vi "graph_diag.vi"(4 "dt":dbl, 6 "Array in":dbl[](array[numeric]), 7 "Averaged":cluster{"xi used":dbl[], "yi":dbl[]}, 9 "DC(V)":dbl, 10 "LD Timetrace in":dbl[][](array[numeric]), 11 "dt":dbl) -> (2 "Time Domain Signal":cluster{"xi used":dbl[], "yi":dbl[]}[](graph), 3 "Spectra":cluster{"f0":dbl, "df":dbl, "magnitude":dbl[]}[](array[cluster]))   [LabVIEW 2013]
uses:
  <vilib>/express/express analysis/Spectral/Block/exnSpectralBlock spectral measurements RMS poly.vi
  <vilib>/express/express analysis/Spectral/Block/exnSpectralBlock spectral measurements RMS WFM.vi
  <vilib>/express/express analysis/Spectral/XNode/ExpressSpectralMeasurementsBlockNode.xnode
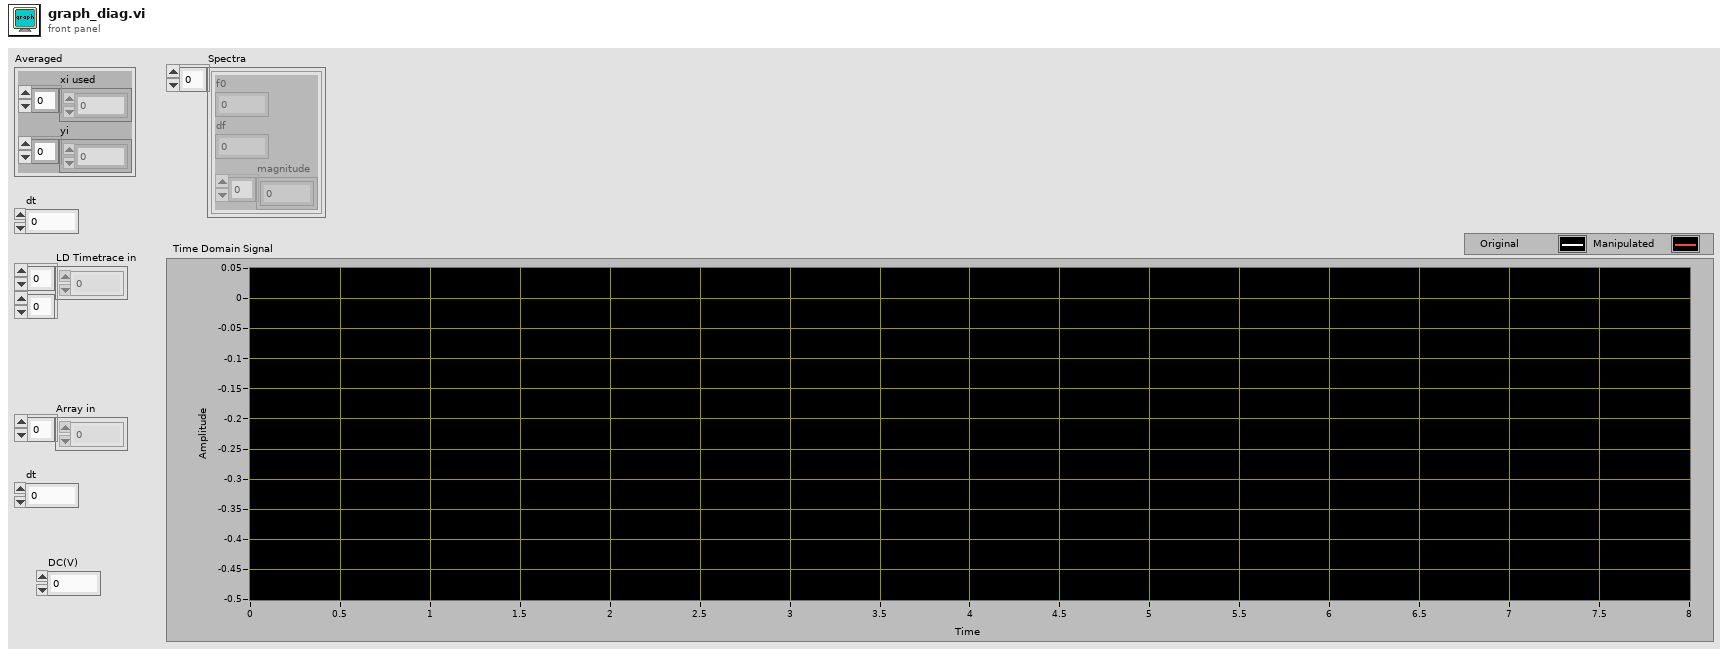
[diagram p1: front panel]
types:
  T1 = cluster{"Array in":dbl[], "LD Timetrace in":dbl[]}
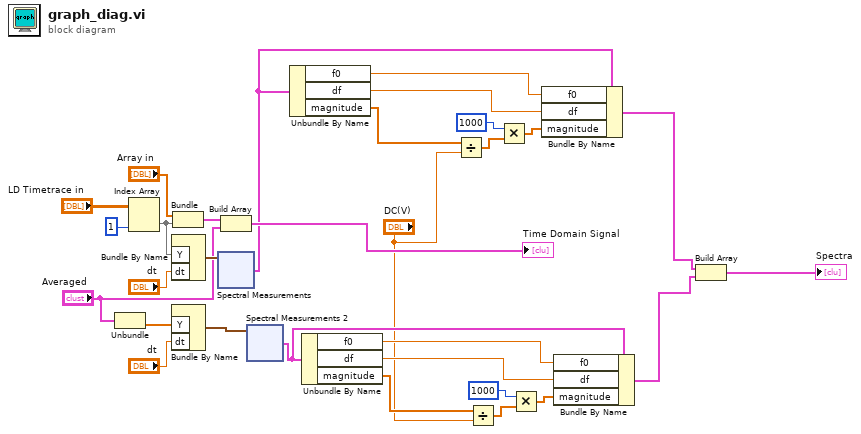
[diagram p0: block diagram]
diagram:
  n1 = Unbundle("Averaged") -> ("yi"=w20:dbl[])  [unwired: 1 out]
  n2 = Index Array(array="LD Timetrace in", index (col)=1 ("disabled index (col)")) -> (element=w24:dbl[])  [unwired: 1 in]
  n3 = Bundle By Name("Y"=w24, "dt"="dt") -> (w23:waveform(dbl))  [unwired: 1 in]
  n4 = Bundle By Name("Y"=w20, "dt"="dt") -> (w25:waveform(dbl))  [unwired: 1 in]
  n5 = Bundle("Array in"="Array in", "LD Timetrace in"=w24) -> (w26:T1)  [unwired: 1 in]
  n6 = xnode "Spectral Measurements"("Signals"=w23) -> ("FFT - (RMS)"=w2:cluster{"f0":dbl, "df":dbl, "magnitude":dbl[]})  [unwired: 1 in, 2 out]
  n7 = Build Array(w26, "Averaged") -> (→"Time Domain Signal":cluster{"xi used":dbl[], "yi":dbl[]}[])
  n8 = xnode "Spectral Measurements 2"("Signals"=w25) -> ("FFT - (RMS)"=w11:cluster{"f0":dbl, "df":dbl, "magnitude":dbl[]})  [unwired: 1 in, 2 out]
  n9 = Unbundle By Name(w2) -> ("f0"=w9:dbl, "df"=w8:dbl, "magnitude"=w6:dbl[])
  n10 = Unbundle By Name(w11) -> ("f0"=w12:dbl, "df"=w13:dbl, "magnitude"=w15:dbl[])
  n11 = Divide(x=w6, y="DC(V)") -> (x/y=w4:dbl[])
  n12 = Divide(x=w15, y="DC(V)") -> (x/y=w17:dbl[])
  n13 = Multiply(x=1000, y=w4) -> (x*y=w7:dbl[])
  n14 = Multiply(x=1000, y=w17) -> (x*y=w14:dbl[])
  n15 = Bundle By Name(cluster=w2, "f0"=w9, "df"=w8, "magnitude"=w7) -> (w3:cluster{"f0":dbl, "df":dbl, "magnitude":dbl[]})
  n16 = Bundle By Name(cluster=w11, "f0"=w12, "df"=w13, "magnitude"=w14) -> (w10:cluster{"f0":dbl, "df":dbl, "magnitude":dbl[]})
  n17 = Build Array(w3, w10) -> (→"Spectra":cluster{"f0":dbl, "df":dbl, "magnitude":dbl[]}[])
